vi "Set Ref Phase Value.vi"(8 "error in (no error)":errorcluster, 10 "Phase Value (0.0 degrees)":dbl format="%.4f", 11 "VISA resource name":refnum<visa-resource-name>) -> (0 "error out":errorcluster, 3 "VISA resource name out":refnum<visa-resource-name>)   [LabVIEW 2014, in "Fluke 5XXX Series Multicalibrators.lvlib"]
doc: "If two Calibrators are synchronized using 10 MHz IN/OUT, sets the phase difference between the primary channel on the Calibrator relative to the sync pulse on the 10 MHz IN or OUT terminal. The primary channel is the NORMAL, AUX, or 20A terminal for single outputs and the NORMAL terminal for ac power and ac dual voltage outputs. The sync pulse on the 10 MHz IN or OUT terminal is the phase reference.\n\nNote:\n\nThis VI is available only for instrument model 5520A."
uses:
  Fluke 5XXX Series Multicalibrators.lvlib
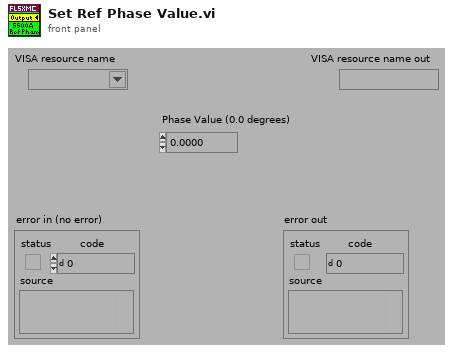
[diagram p1: front panel]
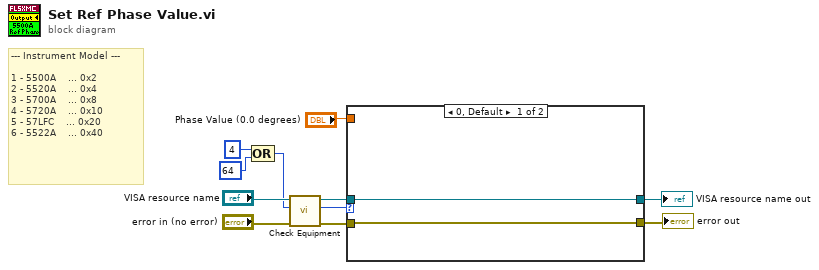
[diagram p0: block diagram]
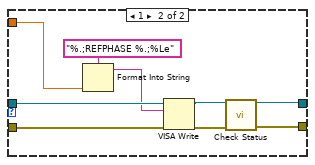
[diagram p2: hidden frame]
diagram:
  # "--- Instrument Model ---\n\n1 - 5500A    ... 0x2\n2 - 5520A    ... 0x4\n3 - 5700A    ... 0x8\n4 - 5720A    ... 0x10\n5 - 57LFC    ... 0x20\n6 - 5522A    ... 0x40"
  n1 = Compound Arithmetic op=OR(4 ("Numeric"), 64 ("Numeric")) -> (w2:i32)
  n2 = call "Check Equipment.vi"("error in (no error)"="error in (no error)", "Bit Mask"=w2, "VISA resource name"="VISA resource name") -> ("error out"=w11:errorcluster, "Present?"=w10:u32, "VISA resource name out"=w9:refnum<visa-resource-name>)  [unwired: 6 in]
  n3 = case shown="0, Default" w10 {
    tunnel: "Phase Value (0.0 degrees)" -> [_ w14]
    tunnel: [w12 w17] -> w4
    tunnel: w11 -> [w13 w22]
    tunnel: w9 -> [w12 w21]
    tunnel: [w13 w20] -> w5
    frame 0, Default {
    }
    frame 1 {
      n4 = Format Into String(format string="%.;REFPHASE %.;%Le", w14) -> (resulting string=w15:string)  [unwired: 2 in, 1 out]
      n5 = VISA Write(VISA resource name=w21, write buffer=w15, error in (no error)=w22) -> (VISA resource name out=w18:refnum<visa-resource-name>, error out=w19:errorcluster)  [unwired: 1 out]
      n6 = call "Check Status.vi"("VISA resource name"=w18, "error in (no error)"=w19) -> ("VISA resource name out"=w17:refnum<visa-resource-name>, "error out"=w20:errorcluster)  [unwired: 12 in]
    }
  }
  "VISA resource name out" <- w4
  "error out" <- w5
